vi "Send.vi"() -> (3 "Destroy Msg out":refnum<class "Destroy Msg.lvclass">)   [LabVIEW 2021, in "Destroy.lvlib" / "Destroy Msg.lvclass"]
uses:
  Destroy Msg.lvclass
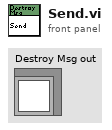
[diagram p1: front panel]
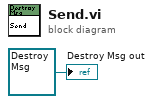
[diagram p0: block diagram]
diagram:
  "Destroy Msg out" <- refnum<class "Destroy Msg.lvclass"> refnum ("Destroy Msg in")
